vi "Get Pressure Module Idn.vi"(8 "error in (no error)":errorcluster, 11 "VISA resource name":refnum<visa-resource-name>) -> (0 "error out":errorcluster, 1 "Model Number":string, 2 "Manufacturer":string, 3 "VISA resource name out":refnum<visa-resource-name>, 4 "Serial Number":string)   [LabVIEW 2014, in "Fluke 5XXX Series Multicalibrators.lvlib"]
doc: "This VI queries the attached pressure module for its model and serial number.\n\nNote:\n\nThis VI is available only for instrument model 5520A with Fluke 700-Pxx external pressure modules."
uses:
  Fluke 5XXX Series Multicalibrators.lvlib
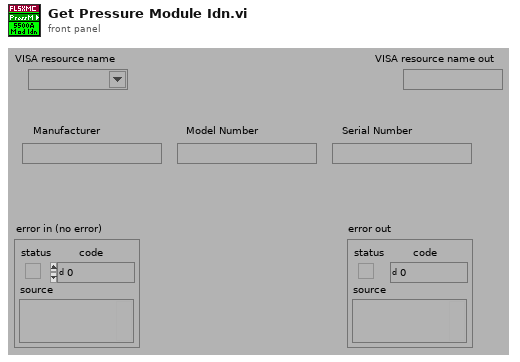
[diagram p1: front panel]
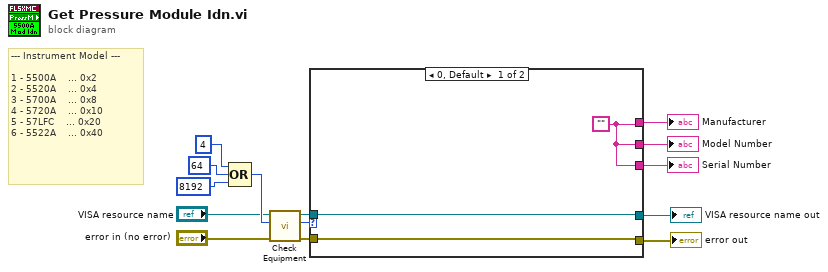
[diagram p0: block diagram]
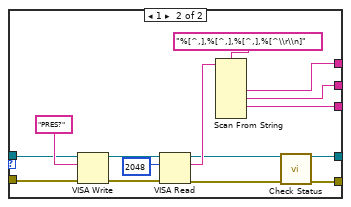
[diagram p2: hidden frame]
diagram:
  # "--- Instrument Model ---\n\n1 - 5500A    ... 0x2\n2 - 5520A    ... 0x4\n3 - 5700A    ... 0x8\n4 - 5720A    ... 0x10\n5 - 57LFC    ... 0x20\n6 - 5522A    ... 0x40"
  n1 = Compound Arithmetic op=OR(4 ("Numeric"), 64 ("Numeric"), 8192 ("Numeric")) -> (w10:i32)
  n2 = call "Check Equipment.vi"("error in (no error)"="error in (no error)", "Bit Mask"=w10, "VISA resource name"="VISA resource name") -> ("error out"=w14:errorcluster, "Present?"=w13:u32, "VISA resource name out"=w12:refnum<visa-resource-name>)  [unwired: 6 in]
  n3 = case shown="0, Default" w13 {
    tunnel: [w17 w22] -> w7
    tunnel: [w16 w21] -> w6
    tunnel: w14 -> [w17 w24]
    tunnel: w12 -> [w16 w23]
    tunnel: [w15 w20] -> w5
    tunnel: [w15 w19] -> w4
    tunnel: [w15 w18] -> w3
    frame 0, Default {
      w15 = ""
    }
    frame 1 {
      n4 = VISA Write(VISA resource name=w23, write buffer="PRES?", error in (no error)=w24) -> (VISA resource name out=w26:refnum<visa-resource-name>, error out=w27:errorcluster)  [unwired: 1 out]
      n5 = VISA Read(VISA resource name=w26, byte count=u32 2048 ("byte count (0)"), error in (no error)=w27) -> (VISA resource name out=w31:refnum<visa-resource-name>, read buffer=w32:string, error out=w30:errorcluster)  [unwired: 1 out]
      n6 = Scan From String(format string="%[^,],%[^,],%[^,],%[^\\r\\n]", input string=w32) -> (output 1=w20:string, output 2=w19:string, output 3=w18:string)  [unwired: 7 in, 3 out]
      n7 = call "Check Status.vi"("VISA resource name"=w31, "error in (no error)"=w30) -> ("VISA resource name out"=w21:refnum<visa-resource-name>, "error out"=w22:errorcluster)  [unwired: 12 in]
    }
  }
  "Manufacturer" <- w5
  "Model Number" <- w4
  "Serial Number" <- w3
  "VISA resource name out" <- w6
  "error out" <- w7
